vi "custom waveform creator.vi"(0 "VISA Refnum in":refnum<visa-resource-name>, 1 "Waveform Name":string, 3 "Channel Name (1)":u16(ring)=1 items=["1"=1, "2"=2, "3"=3, "4"=4], 5 "Waveform Graph 2":dbl[](graph), 7 "Waveform Graph":dbl[](graph), 9 "Periods (1)":dbl=1.0, 11 "error in (no error)":errorcluster, 12 "Frequency (100KHz)":u32=100000, 14 "Samples (1000)":u32=1000) -> (4 "VISA Refnum out":refnum<visa-resource-name>, 15 "error out":errorcluster)   [LabVIEW 2018, in "Tektronix AWG 5000 7000 Series.lvlib"]
uses:
  <instrlib>/Tektronix AWG 5000 7000 Series/Tektronix AWG 5000 7000 Series.lvlib
  <instrlib>/Tektronix AWG 5000 7000 Series/Public/Configure/Channel/Assign Output Waveform (From Waveform List).vi
  <instrlib>/Tektronix AWG 5000 7000 Series/Public/Configure/Configure Output Timing (Repetition Rate).vi
panel:
  out "Waveform Graph 3":dbl[](graph)
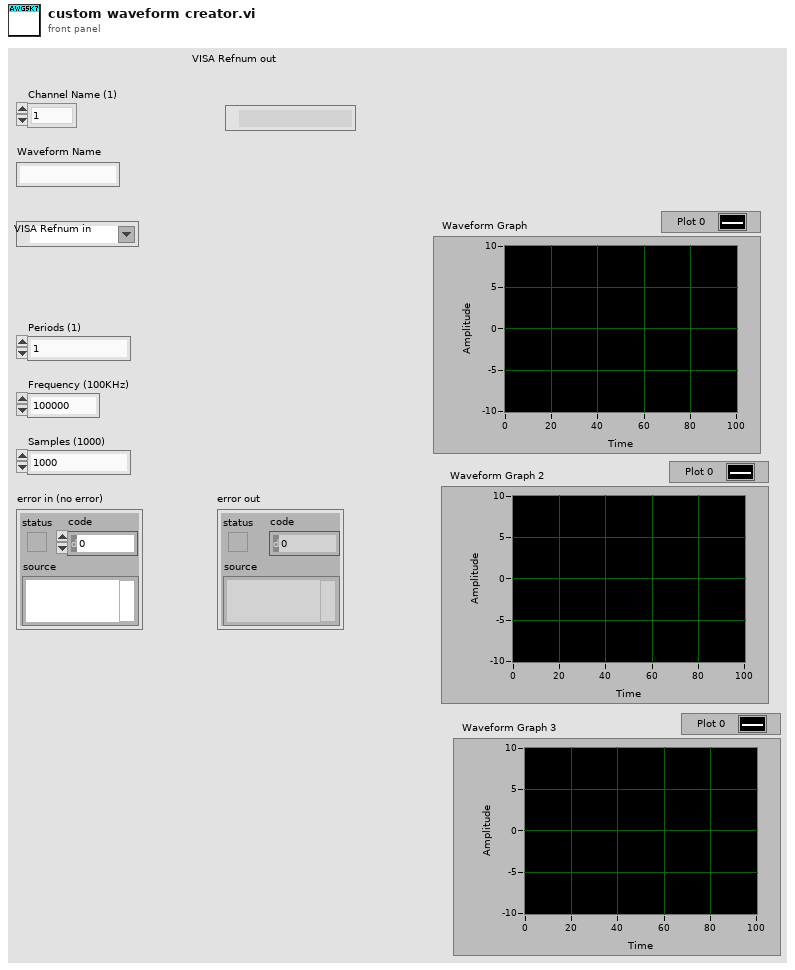
[diagram p1: front panel]
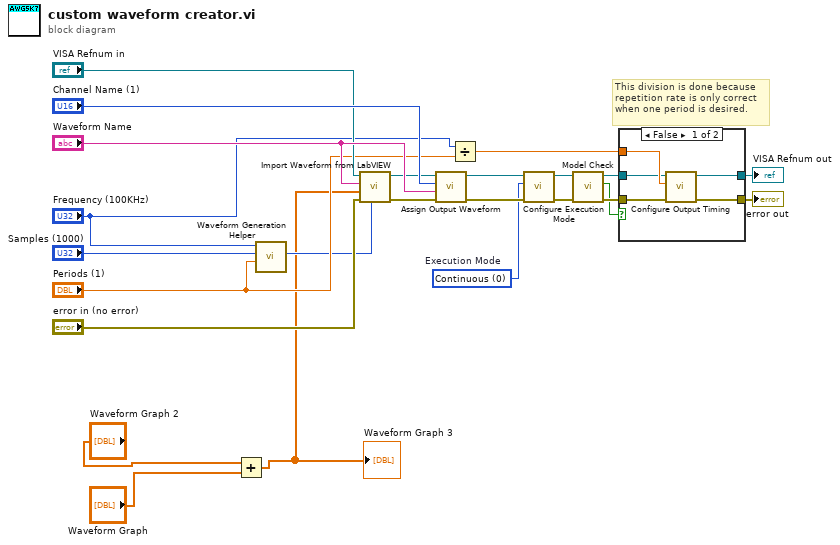
[diagram p0: block diagram]
diagram:
  w11 = u16 0 items=["Continuous", "Triggered", "Gated", "Sequence"]  # Execution Mode
  # "This division is done because\nrepetition rate is only correct\nwhen one period is desired."
  n1 = Add(x="Waveform Graph 2", y="Waveform Graph") -> (x+y=w1:dbl[])
  "Waveform Graph 3" <- w1
  n2 = call <instrlib>:"Waveform Generation Helper.vi"("Period Count (1)"="Periods (1)", "Sample Count (1000)"="Samples (1000)", "Frequency (50KHz)"="Frequency (100KHz)") -> ()  [unwired: 7 in, 2 out]
  n3 = call <instrlib>:"Import Waveform from LabVIEW.vi"("Sample Count (1000)"="Samples (1000)", "error in (no error)"="error in (no error)", "Waveform"=w1, "Waveform Name"="Waveform Name", "VISA resource name"="VISA Refnum in") -> ("error out"=w15:errorcluster, "VISA resource name out"=w14:refnum<visa-resource-name>)  [unwired: 5 in]
  n4 = call-poly <instrlib>:"Assign Output Waveform.vi"("error in (no error)"=w15, "Waveform"="Waveform Name", "Channel Name (1)"="Channel Name (1)", "VISA resource name"=w14) -> ("error out"=w12:errorcluster, "VISA resource name out"=w13:refnum<visa-resource-name>)  [unwired: 6 in]
  n5 = Divide(x="Frequency (100KHz)", y="Periods (1)") -> (x/y=w16:dbl)
  n6 = call <instrlib>:"Configure Execution Mode.vi"("error in (no error)"=w12, "Execution Mode (0 : Continuous)"=w11, "VISA resource name"=w13) -> ("error out"=w19:errorcluster, "VISA resource name out"=w20:refnum<visa-resource-name>)  [unwired: 7 in]
  n7 = call <instrlib>:"Model Check.vi"("error in (no error)"=w19, "VISA resource name"=w20) -> ("error out"=w22:errorcluster, "Is 70000 Series"=w21:bool, "VISA resource name out"=w23:refnum<visa-resource-name>)  [unwired: 7 in]
  n8 = case shown="False" w21 {
    tunnel: [w28 w30] -> w5
    tunnel: [w27 w29] -> w6
    tunnel: w16 -> [w26 _]
    tunnel: w22 -> [w25 w29]
    tunnel: w23 -> [w24 w30]
    frame False {
      n9 = call-poly <instrlib>:"Configure Output Timing.vi"("error in (no error)"=w25, "Repetition Rate (Hz) (10MHz)"=w26, "VISA resource name"=w24) -> ("error out"=w27:errorcluster, "VISA resource name out"=w28:refnum<visa-resource-name>)  [unwired: 7 in]
    }
    frame True {
      # "AWG70000 series"
      # "Not supported"
    }
  }
  "error out" <- w6
  "VISA Refnum out" <- w5
